vi "9093_第2回_山口修平.vi"() -> ()   [LabVIEW 2020]
panel:
  out "残り時間(秒)":dbl
  out "経過時間(秒)":dbl
  out "秒":dbl
  out "10秒":dbl
  out "分":dbl
  out "時":dbl
  in  "指定時間(秒)":dbl
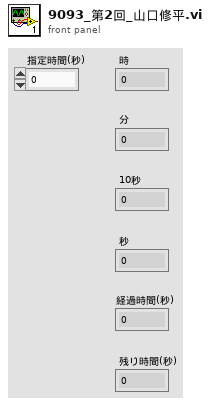
[diagram p1: front panel]
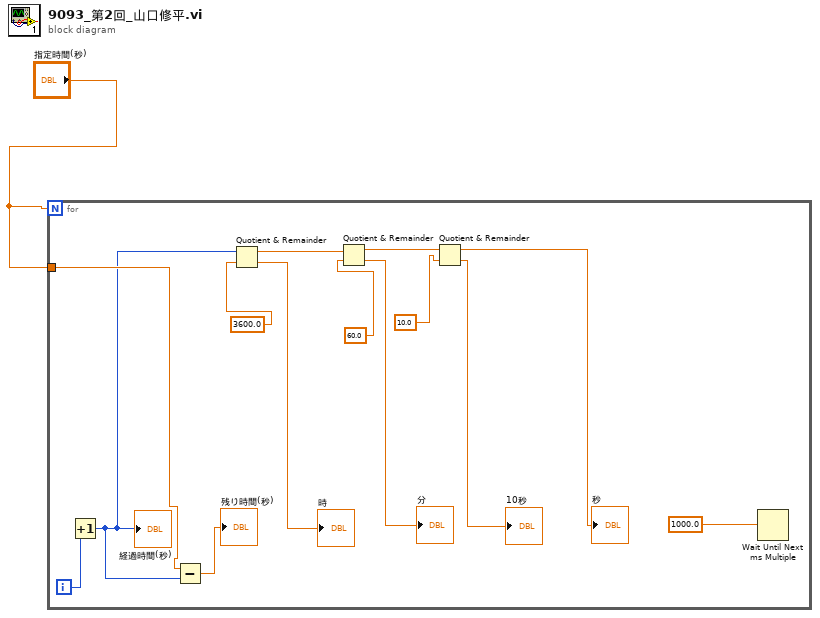
[diagram p0: block diagram]
diagram:
  n1 = for {
    N: "指定時間(秒)" -> [_]
    tunnel: "指定時間(秒)" -> [w13]
    i -> [w14]
    n2 = Increment(x=w14) -> (x+1=w11:i32)
    "経過時間(秒)" <- w11
    n3 = Subtract(x=w13, y=w11) -> (x-y=→"残り時間(秒)":dbl)
    n4 = Quotient & Remainder(x=w11, y=3600.0) -> (x-y*floor(x/y)=w10:dbl, floor(x/y)=→"時":dbl)
    n5 = Quotient & Remainder(x=w10, y=60.0) -> (x-y*floor(x/y)=w9:dbl, floor(x/y)=→"分":dbl)
    n6 = Quotient & Remainder(x=w9, y=10.0) -> (x-y*floor(x/y)=→"秒":dbl, floor(x/y)=→"10秒":dbl)
    n7 = Wait Until Next ms Multiple(millisecond multiple=1000.0) -> ()  [unwired: 1 out]
  }
